vi "Lezeti_Power_Monitor_32_g.vi"() -> ()   [LabVIEW 2014]
uses:
  <vilib>/addons/Electrical Power/Basic/Controls/Vector Diagram/EPX Vector Diagram.xctl
  <vilib>/measure/madcrms.llb/Basic Averaged DC-RMS for N Chan.vi
  <vilib>/measure/madcrms.llb/Basic Averaged DC-RMS for 1 Chan.vi
  <vilib>/addons/Electrical Power/Basic/Measurement/Power (1 Channel).vi
  <vilib>/addons/Electrical Power/Basic/Measurement/Fundamental Vector (N Channels).vi
  <vilib>/Utility/file.llb/Write To Spreadsheet File (DBL).vi
  <vilib>/measure/NI_MAPro.lvlib
  <vilib>/addons/Electrical Power/Basic/NI_EP_Basic.lvlib
panel:
  out "DC Current (Amps)":dbl
  out "DC Voltage":dbl
  out "DC Power (Watts)":dbl
  out "Current Vector":cdb[](array[numeric])
  out "Current Vector Diagram":cdb[](xcontrol)
  out "voltage vector":cdb[](array[numeric])
  out "Voltage Vector Diagram":cdb[](xcontrol)
  out "Reactive Power (VAR) EPS Check 2":dbl
  out "Power Factor EPS Check":dbl
  out "Apparent Power (VA) EPS Check":dbl
  out "Average Power (Watts) EPS Check":dbl
  in  "High Resolution Waveform Data Path":path
  out "Power Factor":dbl
  in  "Average Power Output File":path
  out "Run Date":string
  out "Run Time":string
  out "Elapsed Time (s)":dbl
  out "Apparent Power (VA)":dbl
  out "Average Power (Watts)":dbl
  out "Instantaneous Power Waveform":waveform(dbl)[](graph)
  out "RMS Voltage L1-L2":dbl
  out "L1 RMS Current":dbl
  in  "Burden Resistor (ohms) (1000)":dbl
  in  "CT Ratio (Iout/Iin) (.0003332)":dbl
  in  "Acquire Sample Size (1000)":dbl
  in  "Acquire Rate (Hz) (1000)":dbl
  in  "Acquire Timeout (1000)":dbl
  out "Line 1 Current Waveform":waveform(dbl)[](graph)
  out "Voltage L1-L2":waveform(dbl)[](graph)
  in  "stop":bool
  # "For Lezeti Air Conditioning System (Greenpath Tech)\nBy Matsu Thornton\nJuly 2016"
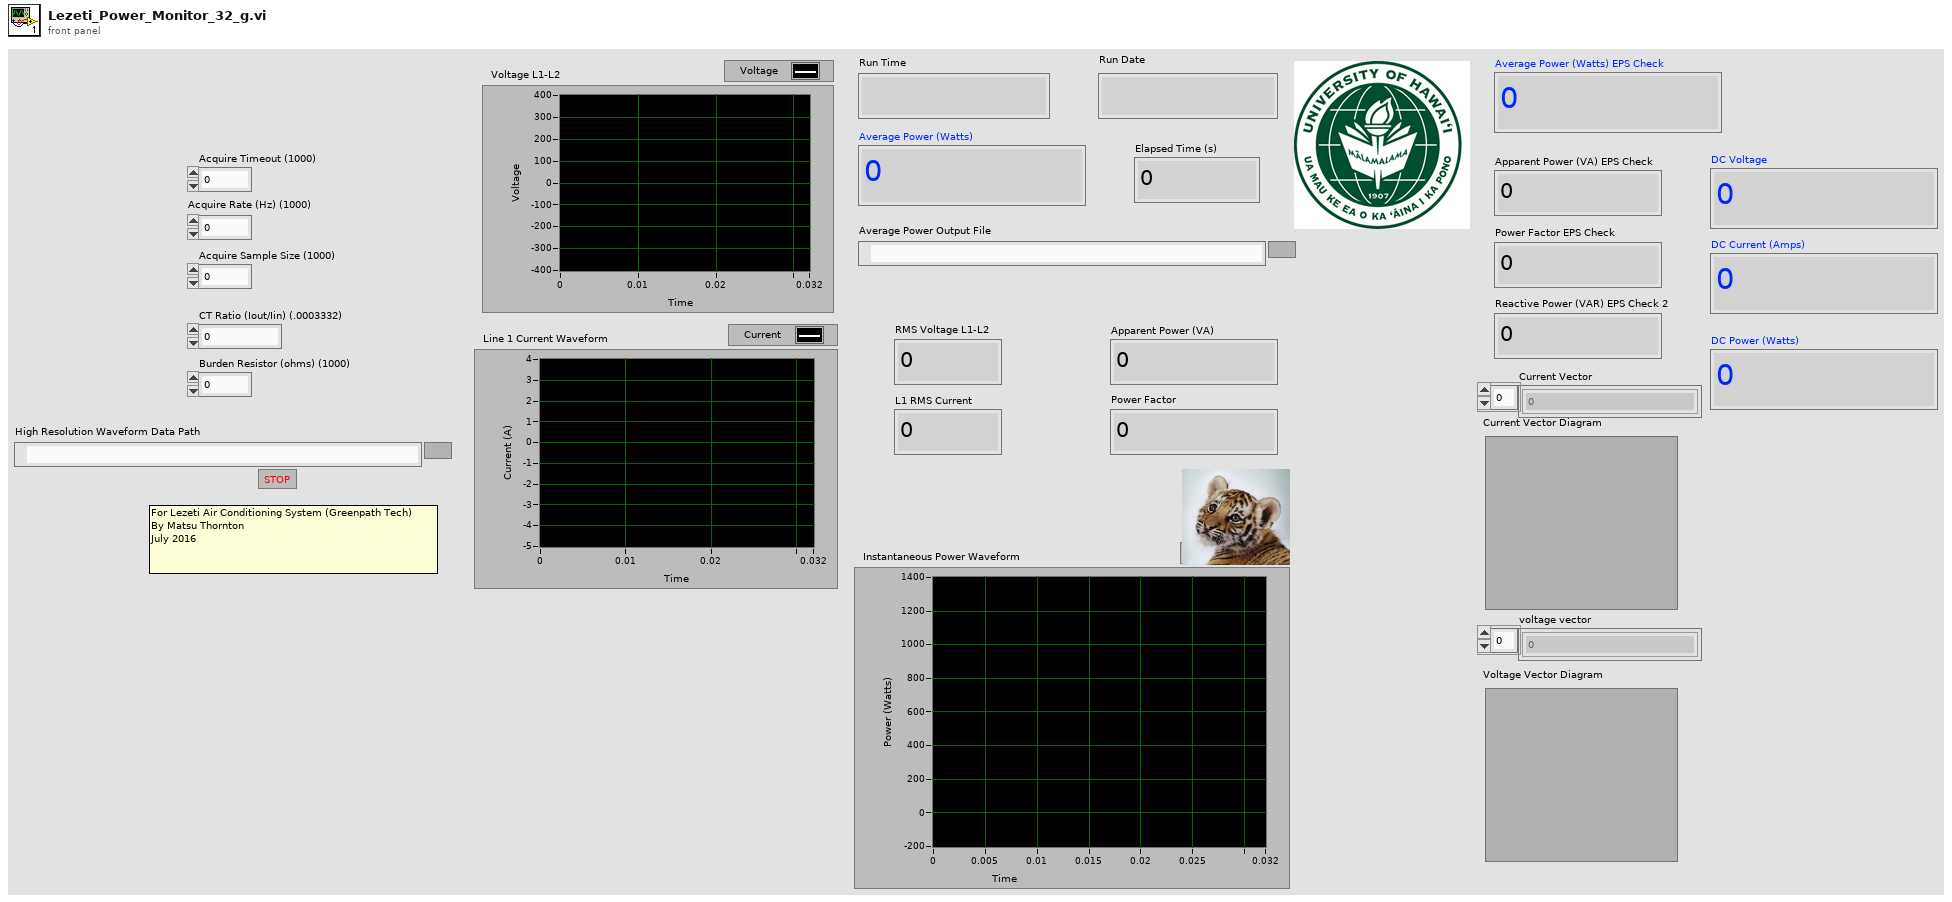
[diagram p1: front panel]
types:
  T1 = typedef "NI_EP_Basic.lvlib/basic_Power Value.ctl" = cluster{"active power [W]":dbl, "apparent power [VA]":dbl, "reactive power [VAR]":dbl, "power factor":dbl}
  T2 = typedef "NI_Matrix.lvlib/RealMatrix.ctl" = dbl[][]
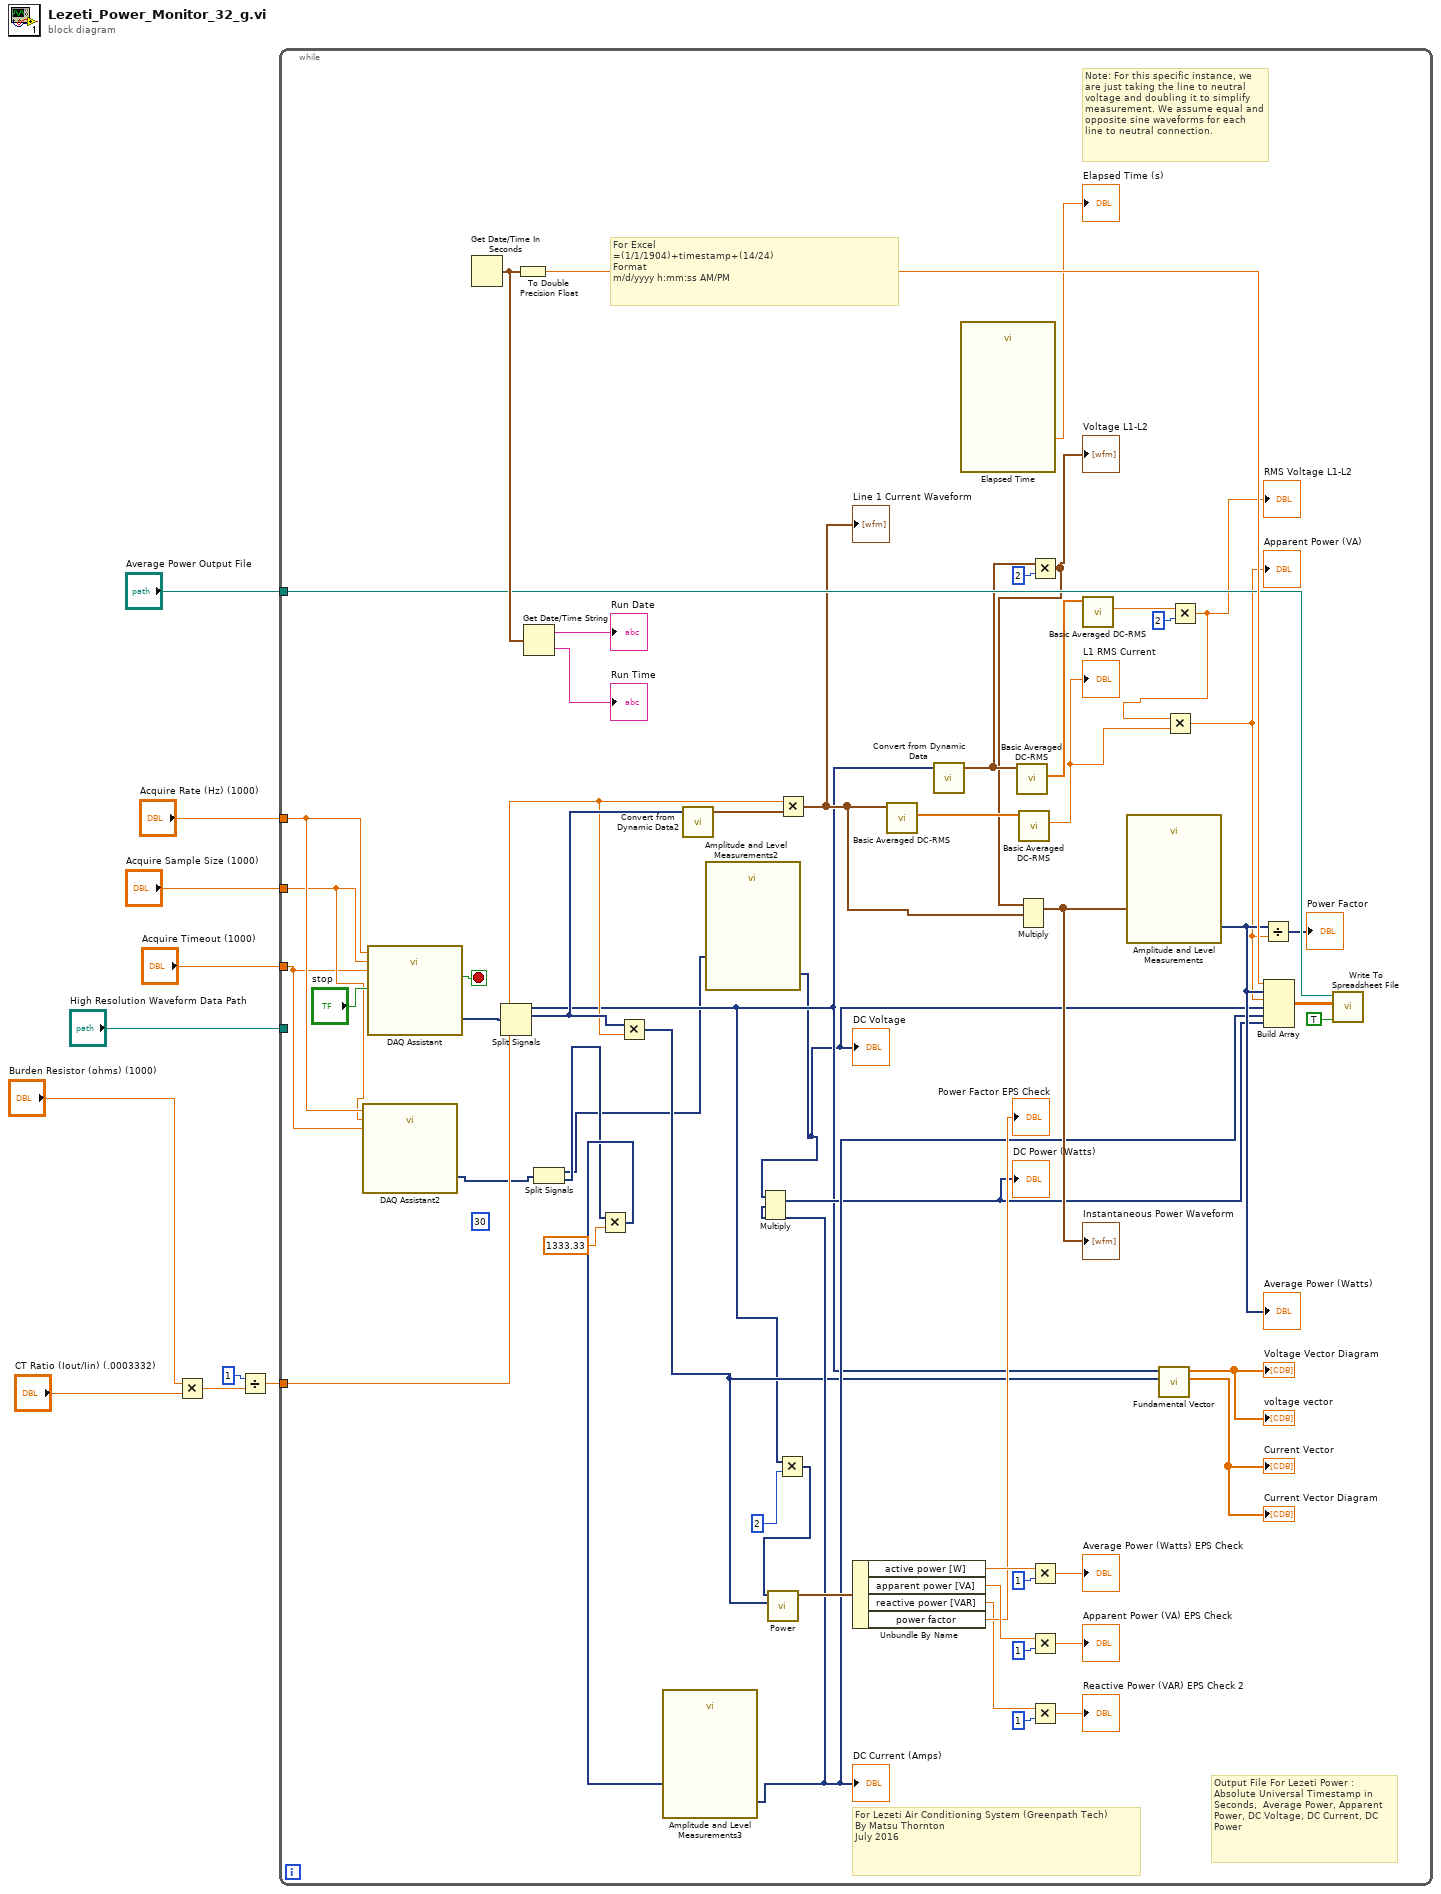
[diagram p0: block diagram]
diagram:
  n1 = Multiply(x="Burden Resistor (ohms) (1000)", y="CT Ratio (Iout/Iin) (.0003332)") -> (x*y=w4:dbl)
  n2 = Divide(x=1, y=w4) -> (x/y=w3:dbl)
  n3 = while {
    tunnel: "Acquire Timeout (1000)" -> [w17]
    tunnel: "Acquire Rate (Hz) (1000)" -> [w19]
    tunnel: "Acquire Sample Size (1000)" -> [w18]
    tunnel: w3 -> [w31]
    tunnel: "Average Power Output File" -> [w55]
    tunnel: "High Resolution Waveform Data Path" -> [_]
    stop <- w52 stop-if-true
    (unwired) 30
    # "Output File For Lezeti Power :\nAbsolute Universal Timestamp in Seconds,  Average Power, Apparent Power, DC Voltage, DC Current, DC Power"
    # "Note: For this specific instance, we are just taking the line to neutral voltage and doubling it to simplify measurement. We assume equal and opposite sine waveforms for each line to neutral connection."
    # "For Excel\n=(1/1/1904)+timestamp+(14/24)\nFormat\nm/d/yyyy h:mm:ss AM/PM"
    # "For Lezeti Air Conditioning System (Greenpath Tech)\nBy Matsu Thornton\nJuly 2016"
    n4 = call "DAQ Assistant2"("rate"=w19, "number of samples"=w18, "timeout (s)"=w17) -> ("data"=w14:dynamicdata)  [unwired: 13 in, 3 out]
    n5 = call "DAQ Assistant"("rate"=w19, "number of samples"=w18, "timeout (s)"=w17, "stop (F)"="stop") -> ("data"=w46:dynamicdata, "stopped"=w52:bool)  [unwired: 12 in, 2 out]
    n6 = Get Date/Time In Seconds() -> (seconds since 1Jan1904=w59:timestamp)
    n7 = Split Signals(w46) -> (w22:dynamicdata, w41:dynamicdata)  [unwired: 4 in, 2 out]
    n8 = To Double Precision Float(number=w59) -> (double precision float=w60:dbl)
    n9 = Get Date/Time String(seconds (now)=w59) -> (date string=→"Run Date":string, time string=→"Run Time":string)  [unwired: 2 in]
    n10 = Split Signals(w14) -> (w12:dynamicdata, w13:dynamicdata)  [unwired: 2 in]
    n11 = Multiply(x=w13, y=1333.33) -> (x*y=w15:dynamicdata)
    n12 = Multiply(x=w41, y=w31) -> (x*y=w24:dynamicdata)
    n13 = call "Amplitude and Level Measurements3"("Signals"=w15) -> ("Mean (DC)"=w30:dynamicdata)  [unwired: 13 in, 1 out]
    "DC Current (Amps)" <- w30
    n14 = call "Convert from Dynamic Data2"("Dynamic Data Type"=w41) -> ("Array of Waveform"=w64:waveform(dbl)[])  [unwired: 3 in]
    n15 = call "Amplitude and Level Measurements2"("Signals"=w12) -> ("Mean (DC)"=w11:dynamicdata)  [unwired: 13 in, 1 out]
    "DC Voltage" <- w11
    n16 = Multiply(1:w30, 2:w11) -> (0:w29:dynamicdata)  [unwired: 1 in, 1 out]
    "DC Power (Watts)" <- w29
    n17 = Multiply(x=w22, y=2) -> (x*y=w21:dynamicdata)
    n18 = call-poly <vilib>:"Power.vi"("current waveform"=w24, "voltage waveform"=w21) -> ("power value"=w45:T1)  [unwired: 8 in, 1 out]
    n19 = Multiply(x=w31, y=w64) -> (x*y=w27:waveform(dbl)[])
    "Line 1 Current Waveform" <- w27
    n20 = Unbundle By Name(w45) -> ("active power [W]"=w43:dbl, "apparent power [VA]"=w38:dbl, "reactive power [VAR]"=w34:dbl, "power factor"=→"Power Factor EPS Check":dbl)
    n21 = call-poly <vilib>:"Basic Averaged DC-RMS.vi"("signals in"=w27) -> ("RMS values"=w65:dbl[])  [unwired: 7 in, 3 out]
    n22 = call "Convert from Dynamic Data"("Dynamic Data Type"=w22) -> ("Array of Waveform"=w47:waveform(dbl)[])  [unwired: 3 in]
    n23 = call "Elapsed Time"() -> ("Elapsed Time (s)"=→"Elapsed Time (s)":dbl)  [unwired: 12 in, 7 out]
    n24 = call-poly <vilib>:"Basic Averaged DC-RMS.vi"("signals in"=w47) -> ("RMS values"=w66:dbl[])  [unwired: 7 in, 3 out]
    n25 = call-poly <vilib>:"Basic Averaged DC-RMS.vi"("signal in"=w65) -> ("RMS value"=w26:dbl)  [unwired: 7 in, 3 out]
    "L1 RMS Current" <- w26
    n26 = Multiply(x=w47, y=2) -> (x*y=w20:waveform(dbl)[])
    "Voltage L1-L2" <- w20
    n27 = Multiply(1:w27, 2:w20) -> (0:w63:waveform(dbl)[])  [unwired: 1 in, 1 out]
    "Instantaneous Power Waveform" <- w63
    n28 = Multiply(x=w43, y=1) -> (x*y=→"Average Power (Watts) EPS Check":dbl)
    n29 = Multiply(x=w38, y=1) -> (x*y=→"Apparent Power (VA) EPS Check":dbl)
    n30 = Multiply(x=w34, y=1) -> (x*y=→"Reactive Power (VAR) EPS Check 2":dbl)
    n31 = call-poly <vilib>:"Basic Averaged DC-RMS.vi"("signal in"=w66) -> ("RMS value"=w49:dbl)  [unwired: 7 in, 3 out]
    n32 = call "Amplitude and Level Measurements"("Signals"=w63) -> ("Mean (DC)"=w54:dynamicdata)  [unwired: 13 in, 1 out]
    "Average Power (Watts)" <- w54
    n33 = call-poly <vilib>:"Fundamental Vector.vi"("current waveforms"=w24, "voltage waveforms"=w22) -> ("current fundamental vectors"=→"Current Vector Diagram" →"Current Vector":cdb[], "voltage fundamental vectors"=→"Voltage Vector Diagram" →"voltage vector":cdb[])  [unwired: 6 in, 2 out]
    n34 = Multiply(x=w49, y=2) -> (x*y=w25:dbl)
    "RMS Voltage L1-L2" <- w25
    n35 = Multiply(x=w25, y=w26) -> (x*y=w51:dbl)
    "Apparent Power (VA)" <- w51
    n36 = Divide(x=w54, y=w51) -> (x/y=→"Power Factor":dynamicdata)
    n37 = Build Array(w60, w54, w51, w11, w30, w29) -> (w61:T2)
    n38 = call-poly <vilib>:"Write To Spreadsheet File.vi"("append to file? (new file:F)"=TRUE, "2D data"=w61, "file path (dialog if empty)"=w55) -> ()  [unwired: 5 in, 1 out]
  }
